vi "Facade.vi"(0 "Data In":T6, 2 "Display State In":T2={"Graph Visible Items"={"Plot Legend"=FALSE, "Scale Legend"=FALSE, "Graph Palette"=FALSE, "Cursor Legend"=FALSE, "X Scrollbar"=FALSE}, "View Table"=FALSE, "Table Visible Items"={"Vertical Scrollbar"=FALSE, "Horizontal Scrollbar"=FALSE, "Row Headers"=FALSE, "Column Headers"=FALSE, "Vertical Lines"=FALSE, "Horizontal Lines"=FALSE}, "Header Font"={"Font Name"="", "Size"=0, "Bold"=FALSE, "Italic"=FALSE, "Underline"=FALSE, "Strikeout"=FALSE, "Color"=0}, "Cell Font"={"Font Name"="", "Size"=0, "Bold"=FALSE, "Italic"=FALSE, "Underline"=FALSE, "Strikeout"=FALSE, "Color"=0}, "Description and Tip..."={"Description"="", "Tip"=""}, "Moveable Splitter Position"=0, "Measurement Cursor Configuration"={"relative to t0"={"enable relative time"=FALSE, "Relative times (DT)"=[], "color"=0}, "range"={"enable range"=FALSE, "T1"=0.0, "T2"=0.0, "Fixed interval (T2-T1)"=0.0, "T1 color"=0, "T2 color"=0, "enable shading"=FALSE}, "periodic"={"enable periodic"=FALSE, "First event (E1)"=0.0, "Number events (Ei)"=0, "Event spacing (s)"=0.0, "First color"=0, "Events color"=0}, "absolute timestamp"={"enable absolute"=FALSE, "Timestamps (TS)"=[], "color"=0}}, "X Increment"=0.0, "X Scale"={"Label Visible"=FALSE, "Label Text"="", "Time Mode"=enum."Relative", "Format String"=""}, "Y Scale"={"Label Visible"=FALSE, "Label Text"="", "Scaling"=enum."Engineering Units", "Format String"=""}, "Colors"={"background"=16777215, "major grid"=8355711, "minor grid"=12632256, "font"=0}, "Cursors"={"List"=[], "Tags"=[]}, "Plots"=[], "Plot Color Wheel"=[3381759, 32768, 982784, 4375295, 13827953, 13457919, 16757522, 4343295, 16728758, 12095254], "registered user events"=variant}, 3 "Container State":T5) -> (6 "Data Out":T6, 7 "Display State Out":T2={"Graph Visible Items"={"Plot Legend"=FALSE, "Scale Legend"=FALSE, "Graph Palette"=FALSE, "Cursor Legend"=FALSE, "X Scrollbar"=FALSE}, "View Table"=FALSE, "Table Visible Items"={"Vertical Scrollbar"=FALSE, "Horizontal Scrollbar"=FALSE, "Row Headers"=FALSE, "Column Headers"=FALSE, "Vertical Lines"=FALSE, "Horizontal Lines"=FALSE}, "Header Font"={"Font Name"="", "Size"=0, "Bold"=FALSE, "Italic"=FALSE, "Underline"=FALSE, "Strikeout"=FALSE, "Color"=0}, "Cell Font"={"Font Name"="", "Size"=0, "Bold"=FALSE, "Italic"=FALSE, "Underline"=FALSE, "Strikeout"=FALSE, "Color"=0}, "Description and Tip..."={"Description"="", "Tip"=""}, "Moveable Splitter Position"=0, "Measurement Cursor Configuration"={"relative to t0"={"enable relative time"=FALSE, "Relative times (DT)"=[], "color"=0}, "range"={"enable range"=FALSE, "T1"=0.0, "T2"=0.0, "Fixed interval (T2-T1)"=0.0, "T1 color"=0, "T2 color"=0, "enable shading"=FALSE}, "periodic"={"enable periodic"=FALSE, "First event (E1)"=0.0, "Number events (Ei)"=0, "Event spacing (s)"=0.0, "First color"=0, "Events color"=0}, "absolute timestamp"={"enable absolute"=FALSE, "Timestamps (TS)"=[], "color"=0}}, "X Increment"=0.0, "X Scale"={"Label Visible"=FALSE, "Label Text"="", "Time Mode"=enum."Relative", "Format String"=""}, "Y Scale"={"Label Visible"=FALSE, "Label Text"="", "Scaling"=enum."Engineering Units", "Format String"=""}, "Colors"={"background"=16777215, "major grid"=8355711, "minor grid"=12632256, "font"=0}, "Cursors"={"List"=[], "Tags"=[]}, "Plots"=[], "Plot Color Wheel"=[3381759, 32768, 982784, 4375295, 13827953, 13457919, 16757522, 4343295, 16728758, 12095254], "registered user events"=variant}, 8 "Action":T1)   [LabVIEW 2017, in "Waveforms with Cursors.xctl"]
doc: "This is the facade VI for the Spectral Graph with Measurement Cursors XControl.\nThe facade VI is only used within the context of the XControl."
uses:
  <vilib>/addons/_XControls/Waveforms with Cursors/Waveforms with Cursors.xctl
  <vilib>/addons/_XControls/Waveforms with Cursors/Controls/Data.ctl
  <vilib>/_xctls/Container State.ctl
  <vilib>/addons/_XControls/Waveforms with Cursors/Controls/State.ctl
  <vilib>/Utility/miscctls.llb/LVFontTypeDef.ctl
  <vilib>/addons/_XControls/Waveforms with Cursors/Controls/Waveform Cursor Configuration.ctl
  <vilib>/_xctls/Action.ctl
  <vilib>/addons/_XControls/Waveforms with Cursors/Controls/Refnums Typedef.ctl
  <vilib>/addons/_XControls/Waveforms with Cursors/Controls/Waveform XControl Events.ctl
  <vilib>/Utility/miscctls.llb/LVForegroundBackgroundColorsTypeDef.ctl
  <vilib>/measure/mamon.llb/Trigger Detection for 1 Channel.vi
  <vilib>/addons/_NISVFA/_Shared subVIs/Groups/SV Get By Measurement Type (sw trigger) (1 Ch).vi
  <vilib>/_xctls/XControlSupport.lvlib
  <vilib>/measure/NI_MAPro.lvlib
panel:
  out "plot names":string[](array[string])
  in  "Focus Boolean":bool
  out "Waveform Graph":waveform(sgl)[](graph)
  in  "View Table":bool=TRUE
  in  "Cursor Table":string[][](table)
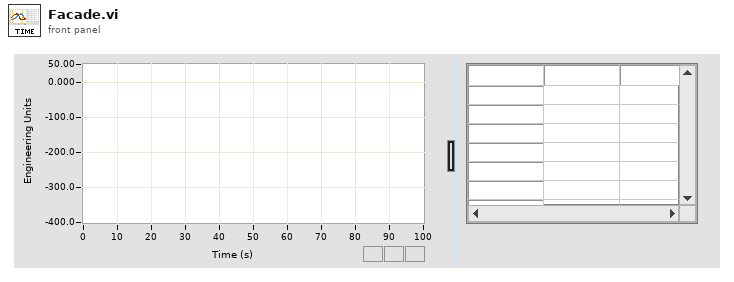
[diagram p1: front panel]
types:
  T1 = typedef "XControlSupport.lvlib/Action.ctl" = cluster{"Data Changed?":bool, "State Changed?":bool, "Action Name":string}
  T2 = typedef "Waveforms with Cursors.xctl/State.ctl" = cluster{"Graph Visible Items":cluster{"Plot Legend":bool, "Scale Legend":bool, "Graph Palette":bool, "Cursor Legend":bool, "X Scrollbar":bool}, "View Table":bool, "Table Visible Items":cluster{"Vertical Scrollbar":bool, "Horizontal Scrollbar":bool, "Row Headers":bool, "Column Headers":bool, "Vertical Lines":bool, "Horizontal Lines":bool}, "Header Font":T3, "Cell Font":T3, "Description and Tip...":cluster{"Description":string, "Tip":string}, "Moveable Splitter Position":i32, "Measurement Cursor Configuration":T4, "X Increment":dbl, "X Scale":cluster{"Label Visible":bool, "Label Text":string, "Time Mode":enum16{"Relative", "Absolute"}, "Format String":string}, "Y Scale":cluster{"Label Visible":bool, "Label Text":string, "Scaling":enum16{"Engineering Units", "Voltage"}, "Format String":string}, "Colors":cluster{"background":u32, "major grid":u32, "minor grid":u32, "font":u32}, "Cursors":cluster{"List":cluster{"Name":string, "Color":u32, "Style":i32, "Point Style":u8, "Name Visible":bool, "Allow Drag":bool, "Cursor Mode":u32, "Plot":i32, "Index":i32, "Position":cluster{"X":dbl, "Y":dbl}, "X Scale":u32, "Y Scale":u32, "Watch Plots":i32[], "Watch All Plots":bool, "Plot Area":i32, "Label Offset":cluster{"X":dbl, "Y":dbl}}[], "Tags":variant[]}, "Plots":cluster{"Name":string, "Line Color":u32, "Line Style":u8, "Line Width":u8, "Fill/Point Color":u32, "Point Style":u8, "Fill To":i16, "Interpolation":u8, "Anti-aliased":bool}[], "Plot Color Wheel":u32[], "registered user events":variant}
  T3 = typedef "LVFontTypeDef.ctl" = cluster{"Font Name":string, "Size":u16, "Bold":bool, "Italic":bool, "Underline":bool, "Strikeout":bool, "Color":u32}
  T4 = typedef "Waveforms with Cursors.xctl/Waveform Cursor Configuration.ctl" = cluster{"relative to t0":cluster{"enable relative time":bool, "Relative times (DT)":dbl[], "color":u32}, "range":cluster{"enable range":bool, "T1":dbl, "T2":dbl, "Fixed interval (T2-T1)":dbl, "T1 color":u32, "T2 color":u32, "enable shading":bool}, "periodic":cluster{"enable periodic":bool, "First event (E1)":dbl, "Number events (Ei)":i32, "Event spacing (s)":dbl, "First color":u32, "Events color":u32}, "absolute timestamp":cluster{"enable absolute":bool, "Timestamps (TS)":timestamp[], "color":u32}}
  T5 = typedef "XControlSupport.lvlib/Container State.ctl" = cluster{"Indicator?":bool, "Run Mode?":bool, " Refnum":refnum<vi>}
  T6 = typedef "Waveforms with Cursors.xctl/Data.ctl" = waveform(dbl)[]
  T7 = typedef "Waveforms with Cursors.xctl/Refnums Typedef.ctl" = cluster{"Splitters":cluster{"Moveable":refnum<vi>, "Locked":refnum<vi>}, "Panes":cluster{"Container":refnum<vi>, "Graph":refnum<vi>, "Table":refnum<vi>, "Fixed-Width":refnum<vi>}, "Controls":cluster{"WFGraph Refnum":refnum<vi>, "Table":refnum<vi>, "View Table":refnum<vi>, "Focus Boolean":refnum<vi>, "Plot Names":refnum<vi>}}
  T8 = typedef "Waveforms with Cursors.xctl/Waveform XControl Events.ctl" = string
  T9 = typedef "LVForegroundBackgroundColorsTypeDef.ctl" = cluster{"Foreground Color":u32, "Background Color":u32}
  T10 = cluster{"level":dbl, "slope":u16, "hysteresis":dbl}
  T11 = typedef "eventvkey.ctl" = enum16{"ASCII", "Enter", "Return", "Shift", "Ctrl", "Alt", "Cmd", "Opt", "Caps", "NumLock", "Clear", "Break", "Up", "Down", "Left", "Right", "Insert", "Delete", "Home", "End", "PageUp", "PageDown", "Escape", "Help", "Pause", "ScrollLock", "F1", "F2", "F3", "F4", "F5", "F6", "F7", "F8", "F9", "F10", "F11", "F12", "F13", "F14", "F15", "F16", "F17", "F18", "F19", "F20", "F21", "F22", "F23", "F24", "Play", "VolumeUp", "VolumeDown", "Mute", "Two Byte Char"}
  T12 = cluster{"Shift":bool, "Ctrl":bool, "Alt":bool, "Cmd":bool, "Opt":bool}
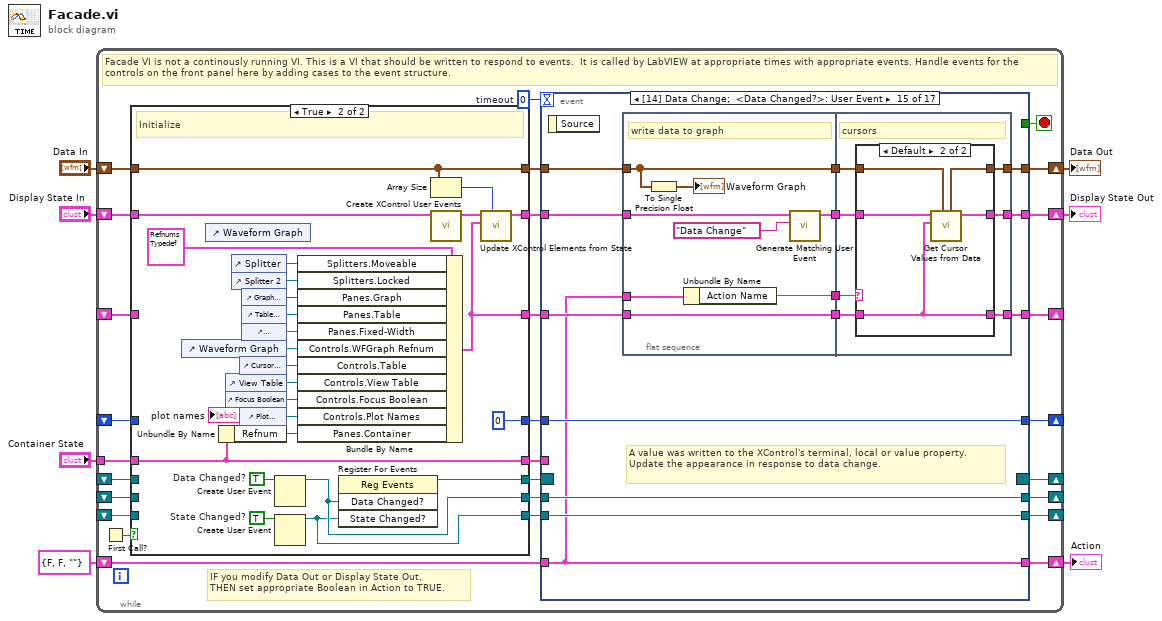
[diagram p0: block diagram]
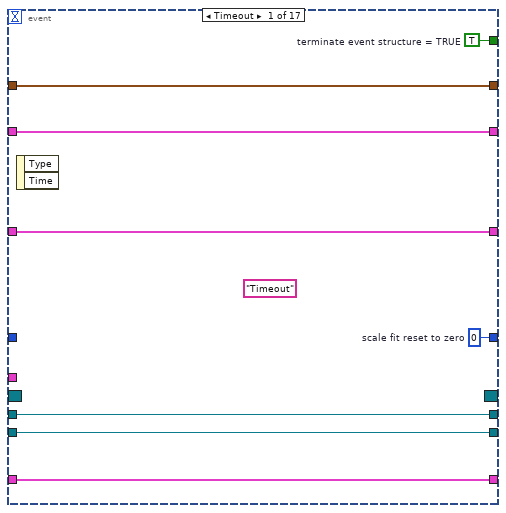
[diagram p3: hidden frame]
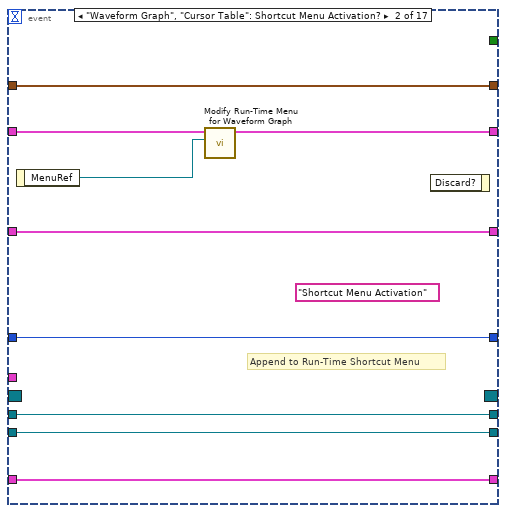
[diagram p4: hidden frame]
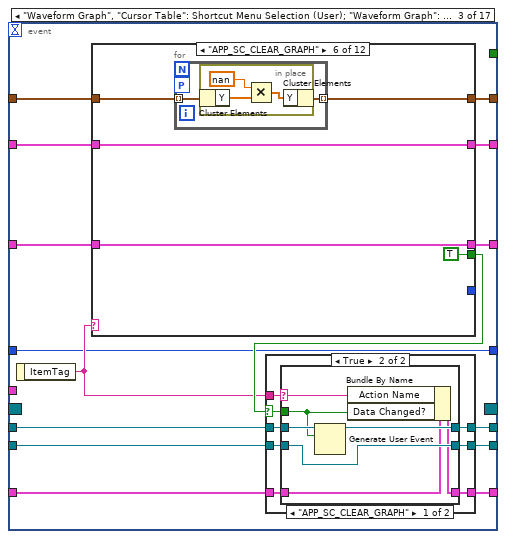
[diagram p5: hidden frame]
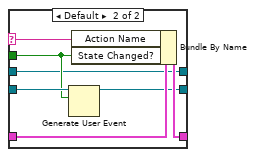
[diagram p7: hidden frame]
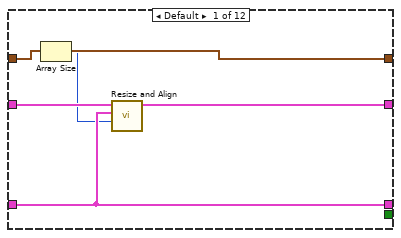
[diagram p8: hidden frame]
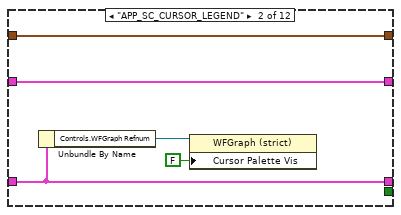
[diagram p9: hidden frame]
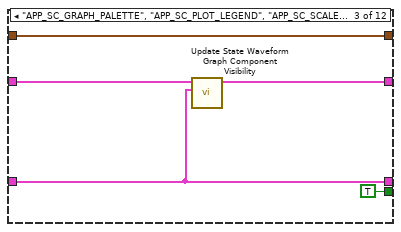
[diagram p10: hidden frame]
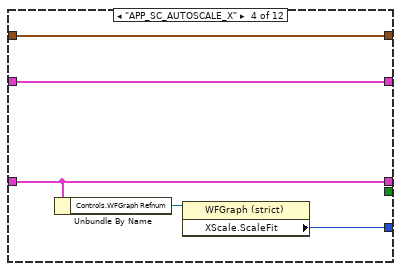
[diagram p11: hidden frame]
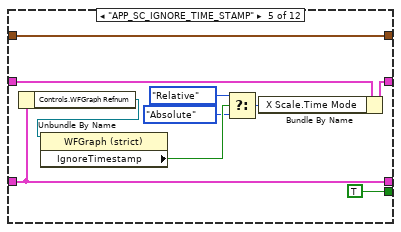
[diagram p12: hidden frame]
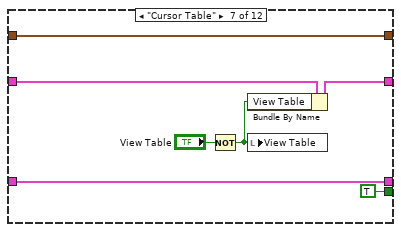
[diagram p13: hidden frame]
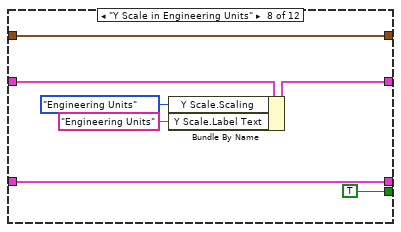
[diagram p14: hidden frame]
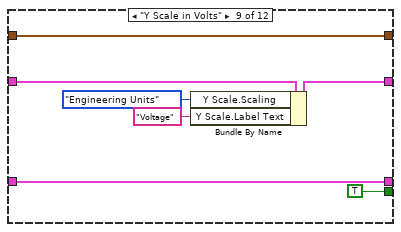
[diagram p15: hidden frame]
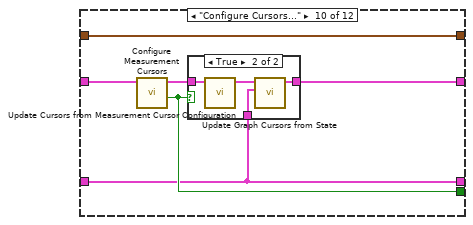
[diagram p16: hidden frame]
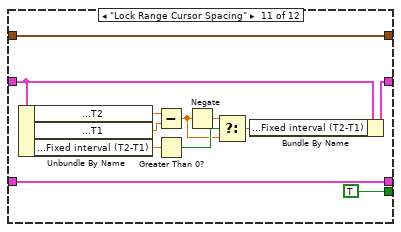
[diagram p18: hidden frame]
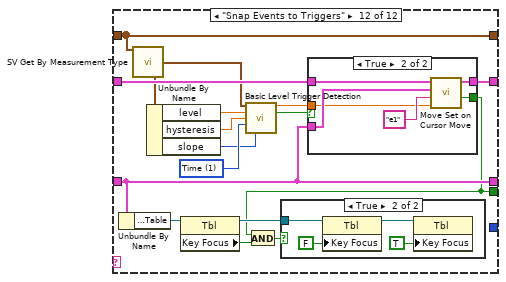
[diagram p19: hidden frame]
diagram:
  n1 = while {
    shift-right: [w15] -> w5
    shift-left: "Display State In" -> [w13]
    tunnel: "Container State" -> [w21]
    shift-right: [w33] -> w7
    shift-left: "Data In" -> [w8]
    shift-right: [w31] -> w2
    shift-left: T1 {"Data Changed?"=FALSE, "State Changed?"=FALSE, "Action Name"=""} ("Action") -> [w32]
    shift-right: [w28] -> _
    shift-left: _ -> [w26]
    shift-right: [w23] -> _
    shift-left: _ -> [w22]
    shift-right: [w27] -> _
    shift-left: _ -> [w24]
    shift-right: [w16] -> _
    shift-left: _ -> [w18]
    shift-right: [w11] -> _
    shift-left: _ -> [w12]
    stop <- w35 stop-if-true
    w34 = 0  # timeout
    # "IF you modify Data Out or Display State Out, \nTHEN set appropriate Boolean in Action to TRUE."
    # "Facade VI is not a continously running VI. This is a VI that should be written to respond to events.  It is called by LabVIEW at appropriate times with appropriate events. Handle events for the controls on the front panel here by adding cases to the event structure."
    n2 = First Call?() -> (First Call?: T/F=w25:bool)
    n3 = case shown="True" w25 {
      tunnel: [w43 w55] -> w17
      tunnel: [w42 w56] -> w30
      tunnel: [w41 w57] -> w29
      tunnel: w26 -> [w43 _]
      tunnel: w24 -> [w42 _]
      tunnel: w22 -> [w41 _]
      tunnel: w21 -> [w39 w51]
      tunnel: [w39 w51] -> w20
      tunnel: [w40 w49] -> w19
      tunnel: w18 -> [w40 _]
      tunnel: [w38 w50] -> w14
      tunnel: w13 -> [w38 w48]
      tunnel: [w37 u8 0 ("Scale Fit")] -> w10
      tunnel: w12 -> [w37 _]
      tunnel: [w36 w45] -> w9
      tunnel: w8 -> [w36 w45]
      frame False {
        # "Continue"
      }
      frame True {
        w68 = TRUE  # State Changed?
        w67 = TRUE  # Data Changed?
        # "Initialize"
        n4 = control-ref of="Waveform Graph"() -> (w63:refnum<vi>)
        n5 = control-ref of="Waveform Graph"() -> ()  [unwired: 1 out]
        n6 = Unbundle By Name(w51) -> ("Refnum"=w53:refnum<vi>)
        n7 = control-ref of="View Table"() -> (w61:refnum<vi>)
        n8 = control-ref of="Focus Boolean"() -> (w54:refnum<vi>)
        n9 = control-ref of="Splitter"() -> (w60:refnum<vi>)
        n10 = control-ref of="Splitter 2"() -> (w59:refnum<vi>)
        n11 = control-ref of="Cursor Table"() -> (w62:refnum<vi>)
        n12 = control-ref of="Plot Names"() -> (w52:refnum<vi>)
        n13 = control-ref of="Graph Pane"() -> (w58:refnum<vi>)
        n14 = control-ref of="Table Pane"() -> (w65:refnum<vi>)
        n15 = control-ref of="Fixed-Width Pane"() -> (w64:refnum<vi>)
        n16 = Create User Event(user event datatype=w67) -> (user event=w57:refnum<user-event>)  [unwired: 1 in, 1 out]
        n17 = Create User Event(user event datatype=w68) -> (user event=w56:refnum<user-event>)  [unwired: 1 in, 1 out]
        n18 = Bundle By Name(cluster=T7 {"Splitters"={"Moveable"=refnum, "Locked"=refnum}, "Panes"={"Container"=refnum, "Graph"=refnum, "Table"=refnum, "Fixed-Width"=refnum}, "Controls"={"WFGraph Refnum"=refnum, "Table"=refnum, "View Table"=refnum, "Focus Boolean"=refnum, "Plot Names"=refnum}} ("Refnums for Resizing and Alignment"), "Splitters.Moveable"=w60, "Splitters.Locked"=w59, "Panes.Graph"=w58, "Panes.Table"=w65, "Panes.Fixed-Width"=w64, "Controls.WFGraph Refnum"=w63, "Controls.Table"=w62, "Controls.View Table"=w61, "Controls.Focus Boolean"=w54, "Controls.Plot Names"=w52, "Panes.Container"=w53) -> (w49:T7)
        n19 = register-events(w57, w56) -> (reference out=w55:refnum<event-registration>)  [unwired: 2 in, 1 out]
        n20 = Array Size(array=w45) -> (size(s)=w44:i32)
        n21 = call <vilib>:"Create XControl User Events.vi"("Display State In in"=w48) -> ("Display State In out"=w47:T2)  [unwired: 9 in, 1 out]
        n22 = call <vilib>:"Update XControl Elements from State.vi"("number of channels"=w44, "Refnums for FP Objects"=w49, "State in"=w47) -> ("State out"=w50:T2)  [unwired: 8 in]
      }
    }
    n23 = event shown="[14] Data Change;  <Data Changed?>: User Event" {
      selector: w17 -> [_ _ _ _ _ _ _ _ _ _ _ _ _ _ _ _ _]
      dyn-events: [_ _ _ _ _ _ _ _ _ _ _ _ _ _ _ _ _] -> w28
      timeout: w34 -> [_ _ _ _ _ _ _ _ _ _ _ _ _ _ _ _ _]
      tunnel: w14 -> [w70 w78 w100 w245 w268 w285 w310 w337 w352 w367 w408 w446 w480 w498 w537 w566 w578]
      tunnel: [w70 w79 w88 w244 w263 w284 w309 w321 w351 w359 w399 w437 w475 w497 w531 w566 w578] -> w15
      tunnel: [w76 _ _ _ _ _ _ _ _ _ _ _ _ _ _ _ _] -> w35
      tunnel: w20 -> [_ _ _ _ _ _ _ _ _ _ _ _ _ _ _ w576 w584]
      tunnel: w9 -> [w74 w85 w90 w238 w272 w302 w319 w338 w356 w377 w417 w455 w485 w487 w535 w575 w583]
      tunnel: [w74 w85 w86 w238 w272 w302 w319 w338 w356 w377 w417 w455 w485 w487 w538 w575 w583] -> w33
      tunnel: [w75 w84 w98 w248 w271 w298 w315 w335 w355 w375 w415 w453 w484 w502 w528 w574 w582] -> w31
      tunnel: w32 -> [w75 w84 w99 w248 w271 w299 w316 w336 w355 w376 w416 w454 w484 w494 w528 w574 w582]
      tunnel: w19 -> [w71 w81 w93 w242 w269 w291 w311 w324 w350 w365 w406 w445 w481 w499 w536 w567 w579]
      tunnel: w29 -> [w73 w83 w94 w246 w265 w297 w314 w330 w353 w371 w411 w449 w482 w501 w540 w571 w581]
      tunnel: w30 -> [w72 w82 w97 w247 w264 w296 w313 w333 w354 w374 w414 w452 w483 w488 w539 w570 w580]
      tunnel: [w72 w82 w96 w247 w264 w295 w312 w332 w354 w373 w413 w451 w483 w489 w539 w570 w580] -> w27
      tunnel: [w73 w83 w95 w246 w265 w297 w314 w331 w353 w372 w412 w450 w482 w500 w540 w571 w581] -> w23
      tunnel: [w71 w81 w92 w243 w269 w291 w311 w324 w350 w365 w406 w445 w481 w495 w530 w567 w579] -> w16
      tunnel: [w69 w77 w87 w239 w261 w281 w307 w320 w349 w357 w398 w436 w474 w491 w529 w565 w577] -> w11
      tunnel: w10 -> [_ w77 w87 _ w262 w281 w307 w320 w349 w357 w398 w436 w474 w491 w529 w565 w577]
      event Timeout {
        w69 = u8 0  # scale fit reset to zero
        (unwired) "Timeout"
        w76 = TRUE  # terminate event structure = TRUE
        n24 = event-data() -> ()  [unwired: 1 in, 2 out]
      }
      event "Waveform Graph", "Cursor Table": Shortcut Menu Activation? {
        (unwired) "Shortcut Menu Activation"
        # "Append to Run-Time Shortcut Menu"
        n25 = event-data() -> ("MenuRef"=w80:refnum<k9>)  [unwired: 1 in]
        n26 = call <vilib>:"Modify Run-Time Menu for Waveform Graph.vi"("Menu in"=w80, "Display State In"=w78) -> ("Display State out"=w79:T2)  [unwired: 9 in]
        n27 = event-data() -> ()  [unwired: 2 in, 1 out]
      }
      event "Waveform Graph", "Cursor Table": Shortcut Menu Selection (User); "Waveform Graph": Shortcut Menu Selection (App) {
        n28 = event-data() -> ("ItemTag"=w89:string)  [unwired: 1 in]
        n29 = case shown="\"APP_SC_CLEAR_GRAPH\"" w89 {
          tunnel: w100 -> [w130 w135 w139 w145 w154 w160 w170 w176 w183 w192 w208 w225]
          tunnel: [w129 w135 w138 w145 w153 w160 w169 w175 w182 w190 w207 w226] -> w88
          tunnel: [_ _ TRUE ("state changed") _ TRUE ("state changed") TRUE ("state changed") TRUE ("state changed") TRUE ("state changed") TRUE ("state changed") w189 TRUE ("state changed") w219] -> w91
          tunnel: w93 -> [w128 w133 w137 w144 w152 w159 w172 w178 w185 w188 w209 w224]
          tunnel: [w128 w133 w137 w144 w152 w159 w172 w178 w185 w188 w209 w224] -> w92
          tunnel: w90 -> [w127 w134 w136 w141 w146 w158 w166 w173 w180 w187 w198 w218]
          tunnel: [_ _ _ w142 _ _ _ _ _ _ _ _] -> _
          tunnel: [w127 w134 w136 w141 w146 w157 w166 w173 w180 w187 w198 w218] -> w86
          frame Default {
            n30 = Array Size(array=w127) -> (size(s)=w126:i32)
            n31 = call <vilib>:"Resize and Align.vi"("number of channels"=w126, "Refnums for Resizing and Alignment"=w128, "State in"=w130) -> ("State out"=w129:T2)  [unwired: 7 in, 1 out]
          }
          frame "APP_SC_CURSOR_LEGEND" {
            n32 = Unbundle By Name(w133) -> ("Controls.WFGraph Refnum"=w132:refnum<vi>)
            n33 = property class="WFGraph (strict)"(reference=w132, "Cursor Palette Vis"=FALSE ("Cursor Legend Visible")) -> ()  [unwired: 1 in, 2 out]
          }
          frame "APP_SC_GRAPH_PALETTE", "APP_SC_PLOT_LEGEND", "APP_SC_SCALE_LEGEND", "APP_SC_X_SCALE", "APP_SC_X_SCROLLBAR", "APP_SC_Y_SCALE" {
            n34 = call <vilib>:"Update State Waveform Graph Component Visibility.vi"("Refnums for FP Objects"=w137, "State in"=w139) -> ("State out"=w138:T2)  [unwired: 9 in]
          }
          frame "APP_SC_AUTOSCALE_X" {
            n35 = Unbundle By Name(w144) -> ("Controls.WFGraph Refnum"=w143:refnum<vi>)
            n36 = property class="WFGraph (strict)"(reference=w143) -> ("XScale.ScaleFit"=w142:u8)  [unwired: 1 in, 2 out]
          }
          frame "APP_SC_IGNORE_TIME_STAMP" {
            n37 = Unbundle By Name(w152) -> ("Controls.WFGraph Refnum"=w151:refnum<vi>)
            n38 = property class="WFGraph (strict)"(reference=w151) -> ("IgnoreTimestamp"=w150:bool)  [unwired: 1 in, 2 out]
            n39 = Select(t=enum16{"Relative", "Absolute"}."Relative" ("X Scale.Time Mode"), s=w150, f=enum16{"Relative", "Absolute"}."Absolute") -> (s? t:f=w147:enum16{"Relative", "Absolute"})
            n40 = Bundle By Name(cluster=w154, "X Scale.Time Mode"=w147) -> (w153:T2)
          }
          frame "APP_SC_CLEAR_GRAPH" {
            n41 = for {
              tunnel: w158 -> [w162] mode=indexing
              tunnel: [w161] -> w157 mode=indexing
              workers-P: _ -> [_]
              n42 = in-place {
                n43 = in-place-cluster #1(w162) -> ("Y"=w164:dbl[])
                n44 = Multiply(x=nan, y=w164) -> (x*y=w163:dbl[])
                n45 = in-place-cluster #1("Y"=w163) -> (w161:waveform(dbl))
              }
            }
          }
          frame "Cursor Table" {
            n46 = Not(x="View Table") -> (.not. x?=w168:bool)
            n47 = Bundle By Name(cluster=w170, "View Table"=w168) -> (w169:T2)
            n48 = local write "View Table"(w168) -> ()
          }
          frame "Y Scale in Engineering Units" {
            n49 = Bundle By Name(cluster=w176, "Y Scale.Scaling"=enum16{"Engineering Units", "Voltage"}."Engineering Units", "Y Scale.Label Text"="Engineering Units") -> (w175:T2)
          }
          frame "Y Scale in Volts" {
            n50 = Bundle By Name(cluster=w183, "Y Scale.Scaling"=enum16{"Engineering Units", "Voltage"}."Engineering Units", "Y Scale.Label Text"="Voltage") -> (w182:T2)
          }
          frame "Configure Cursors..." {
            n51 = call <vilib>:"Configure Measurement Cursors.vi"("State in"=w192) -> ("OK"=w189:bool, "State out"=w191:T2)  [unwired: 9 in]
            n52 = case shown="True" w189 {
              tunnel: w191 -> [w193 w197]
              tunnel: [w193 w195] -> w190
              tunnel: w188 -> [_ w194]
              frame False {
              }
              frame True {
                n53 = call <vilib>:"Update Cursors from Measurement Cursor Configuration.vi"("State in"=w197) -> ("State out"=w196:T2)  [unwired: 10 in]
                n54 = call <vilib>:"Update Graph Cursors from State.vi"("Refnums for FP Objects"=w194, "State in"=w196) -> ("State out"=w195:T2)  [unwired: 9 in]
              }
            }
          }
          frame "Lock Range Cursor Spacing" {
            n55 = Unbundle By Name(w208) -> ("Measurement Cursor Configuration.range.T2"=w206:dbl, "Measurement Cursor Configuration.range.T1"=w205:dbl, "Measurement Cursor Configuration.range.Fixed interval (T2-T1)"=w204:dbl)
            n56 = Subtract(x=w206, y=w205) -> (x-y=w200:dbl)
            n57 = Greater Than 0?(x=w204) -> (x > 0?=w203:bool)
            n58 = Negate(x=w200) -> (-x=w202:dbl)
            n59 = Select(t=w202, s=w203, f=w200) -> (s? t:f=w201:dbl)
            n60 = Bundle By Name(cluster=w208, "Measurement Cursor Configuration.range.Fixed interval (T2-T1)"=w201) -> (w207:T2)
          }
          frame "Snap Events to Triggers" {
            w215 = u16 1 items=["Index", "Time"] ("location mode")
            n61 = Unbundle By Name(w224) -> ("Controls.Table"=w223:refnum<vi>)
            n62 = call-poly <vilib>:"SV Get By Measurement Type.vi"("scaled signals [EU]"=w218) -> ("trigger channel"=w217:waveform(dbl), "level trigger configuration"=w213:T10)  [unwired: 8 in, 5 out]
            n63 = Unbundle By Name(w213) -> ("level"=w212:dbl, "hysteresis"=w211:dbl, "slope"=w210:u16)
            n64 = property class="Tbl"(reference=w223) -> (reference out=w222:refnum<vi>, "Key Focus"=w221:bool)  [unwired: 1 in, 1 out]
            n65 = call-poly <vilib>:"Basic Level Trigger Detection.vi"("signal in"=w217, "level"=w212, "hysteresis"=w211, "location mode"=w215, "trigger slope"=w210) -> ("trigger location"=w214:dbl, "trigger detected?"=w216:bool)  [unwired: 8 in, 1 out]
            n66 = case shown="True" w216 {
              tunnel: [w231 w237] -> w226
              tunnel: w225 -> [w231 w236]
              tunnel: w224 -> [_ w235]
              tunnel: [_ w233] -> w219
              tunnel: w214 -> [_ w232]
              frame False {
              }
              frame True {
                n67 = call <vilib>:"Move Set on Cursor Move.vi"("Cursor.Position.X"=w232, "Cursor Name"="e1", "Refnums for Resizing and Alignment"=w235, "Display State In"=w236) -> ("state changed"=w233:bool, "Display State Out"=w237:T2)  [unwired: 6 in]
              }
            }
            n68 = And(x=w219, y=w221) -> (x .and. y?=w220:bool)
            n69 = case shown="True" w220 {
              tunnel: w222 -> [_ w229]
              frame False {
              }
              frame True {
                n70 = property class="Tbl"(reference=w229, "Key Focus"=FALSE) -> (reference out=w228:refnum<vi>)  [unwired: 1 in, 1 out]
                n71 = property class="Tbl"(reference=w228, "Key Focus"=TRUE) -> ()  [unwired: 1 in, 2 out]
              }
            }
          }
        }
        n72 = case shown="True" w91 {
          selector: w91 -> [_ w107]
          tunnel: w99 -> [w103 w111]
          tunnel: [w103 w110] -> w98
          tunnel: w89 -> [_ w106]
          tunnel: w97 -> [w102 w109]
          tunnel: [w102 w108] -> w96
          tunnel: [w101 w105] -> w95
          tunnel: w94 -> [w101 w104]
          frame False {
          }
          frame True {
            n73 = case shown="\"APP_SC_CLEAR_GRAPH\"" w106 {
              selector: w106 -> [w112 w120]
              tunnel: w111 -> [w114 w125]
              tunnel: [w113 w124] -> w110
              tunnel: w109 -> [w118 w123]
              tunnel: [w118 w122] -> w108
              tunnel: w107 -> [w115 w121]
              tunnel: [w116 w119] -> w105
              tunnel: w104 -> [w117 w119]
              frame "APP_SC_CLEAR_GRAPH" {
                n74 = Generate User Event(user event=w117, event data cluster=w115) -> (user event out=w116:refnum<user-event>)  [unwired: 2 in, 1 out]
                n75 = Bundle By Name(cluster=w114, "Action Name"=w112, "Data Changed?"=w115) -> (w113:T1)
              }
              frame Default {
                n76 = Generate User Event(user event=w123, event data cluster=w121) -> (user event out=w122:refnum<user-event>)  [unwired: 2 in, 1 out]
                n77 = Bundle By Name(cluster=w125, "Action Name"=w120, "State Changed?"=w121) -> (w124:T1)
              }
            }
          }
        }
      }
      event "Waveform Graph": Autoscale Range Change {
        n78 = event-data() -> ("Kind"=w240:enum16{"X-Scale", "Y-Scale", "Z-Scale"}, "ScaleRef"=w241:refnum<vi>)  [unwired: 1 in]
        n79 = property class="GrphScl"(reference=w241) -> ("ScaleFit"=w239:u8)  [unwired: 1 in, 2 out]
        n80 = case shown="\"Y-Scale\"" w240 {
          tunnel: w245 -> [w250 w255]
          tunnel: [w250 w254] -> w244
          tunnel: [w249 w253] -> w243
          tunnel: w242 -> [w249 w252]
          tunnel: w239 -> [_ w251]
          frame "X-Scale", Default {
          }
          frame "Y-Scale" {
            n81 = case shown="1, 2" w251 {
              tunnel: w255 -> [w257 w260]
              tunnel: w252 -> [w256 w258]
              tunnel: [w257 w259] -> w254
              tunnel: [w256 w258] -> w253
              frame 0, Default {
                # "YScaleFit\nManual"
              }
              frame 1, 2 {
                # "YScaleFit\nAuto"
                n82 = call <vilib>:"Adjust Cursor Y Position to Maintain Label Placement.vi"("Refnums for Resizing and Alignment"=w258, "Display State In"=w260) -> ("Display State Out"=w259:T2)  [unwired: 9 in]
              }
            }
          }
        }
      }
      event "Waveform Graph": Scale Range Change {
        (unwired) "Scale Range Change"
        # "this tells us if the scale range changed due to autoscale being set"
        n83 = event-data() -> ("Kind"=w267:enum16{"X-Scale", "Y-Scale", "Z-Scale"}, "ScaleRef"=w270:refnum<vi>)  [unwired: 1 in]
        n84 = case shown="0" w262 {
          selector: w262 -> [_ w274]
          tunnel: w270 -> [_ w276]
          tunnel: [_ w275] -> w266
          tunnel: [u8 0 ("Scale Fit") w274] -> w261
          frame Default {
          }
          frame 0 {
            n85 = property class="GrphScl"(reference=w276, "ScaleFit"=w274) -> (error out=w275:errorcluster)  [unwired: 1 in, 1 out]
          }
        }
        n86 = case shown="\"Y-Scale\"" w267 {
          tunnel: w269 -> [_ w280]
          tunnel: w268 -> [w277 w279]
          tunnel: [w277 w278] -> w263
          tunnel: w266 -> [_ _]
          frame Default {
          }
          frame "Y-Scale" {
            n87 = call <vilib>:"Adjust Cursor Y Position to Maintain Label Placement.vi"("Refnums for Resizing and Alignment"=w280, "Display State In"=w279) -> ("Display State Out"=w278:T2)  [unwired: 9 in]
          }
        }
      }
      event Pane Size {
        w293 = 10  # width - hidden splitter position
        w300 = TRUE
        n88 = event-data() -> ()  [unwired: 1 in, 6 out]
        n89 = Unbundle By Name(w291) -> ("Panes.Container"=w289:refnum<vi>, "Splitters.Moveable"=w290:refnum<vi>)
        n90 = property class="Ctl"(reference=w289) -> ("Width"=w294:u32)  [unwired: 1 in, 2 out]
        n91 = property class="Splitter"(reference=w290) -> ("Position"=w282:i32)  [unwired: 1 in, 2 out]
        n92 = Generate User Event(user event=w296, event data cluster=w300) -> (user event out=w295:refnum<user-event>)  [unwired: 2 in, 1 out]
        n93 = To Long Integer(number=w294) -> (32bit integer=w292:i32)
        n94 = Bundle By Name(cluster=w299, "Action Name"="Resize", "State Changed?"=w300) -> (w298:T1)
        n95 = Unbundle By Name(w285) -> ("View Table"=w286:bool)
        n96 = Subtract(x=w292, y=w293) -> (x-y=w288:i32)
        n97 = Not Equal?(x=w288, y=w282) -> (x != y?=w287:bool)
        n98 = And(x=w286, y=w287) -> (x .and. y?=w283:bool)
        n99 = case shown="True" w283 {
          tunnel: w285 -> [w303 w306]
          tunnel: [w303 w305] -> w284
          tunnel: w282 -> [_ w304]
          frame False {
          }
          frame True {
            n100 = Bundle By Name(cluster=w306, "Moveable Splitter Position"=w304) -> (w305:T2)
          }
        }
      }
      event "View Table": Value Change {
        w317 = TRUE
        n101 = event-data() -> ("NewVal"=w308:bool)  [unwired: 1 in]
        n102 = Bundle By Name(cluster=w310, "View Table"=w308) -> (w309:T2)
        n103 = Generate User Event(user event=w313, event data cluster=w317) -> (user event out=w312:refnum<user-event>)  [unwired: 2 in, 1 out]
        n104 = Bundle By Name(cluster=w316, "Action Name"="View Table Value Change", "State Changed?"=w317) -> (w315:T1)
      }
      event "Waveform Graph": Cursor Move; "Waveform Graph": Cursor Grab {
        n105 = event-data() -> ("CursRef"=w328:refnum<vi>, "CursLoc"=w329:cluster{"X":dbl, "Y":dbl})  [unwired: 1 in]
        n106 = property class="Curs"(reference=w328) -> ("Cursor Name"=w327:string)  [unwired: 1 in, 2 out]
        n107 = Unbundle By Name(w329) -> ("X"=w326:dbl)
        n108 = call <vilib>:"Move Set on Cursor Move.vi"("Cursor.Position.X"=w326, "Cursor Name"=w327, "Refnums for Resizing and Alignment"=w324, "Display State In"=w337) -> ("state changed"=w325:bool, "Display State Out"=w321:T2)  [unwired: 6 in]
        n109 = Unbundle By Name(w324) -> ("Controls.Focus Boolean"=w323:refnum<vi>)
        n110 = case shown="True" w325 {
          selector: w325 -> [_ w344]
          tunnel: w336 -> [w341 w348]
          tunnel: [w341 w347] -> w335
          tunnel: "Cursor Move" -> [_ w346]
          tunnel: w333 -> [w340 w345]
          tunnel: [w340 w343] -> w332
          tunnel: [w339 w342] -> w331
          tunnel: w330 -> [w339 w342]
          frame False {
          }
          frame True {
            n111 = Generate User Event(user event=w345, event data cluster=w344) -> (user event out=w343:refnum<user-event>)  [unwired: 2 in, 1 out]
            n112 = Bundle By Name(cluster=w348, "Action Name"=w346, "State Changed?"=w344) -> (w347:T1)
          }
        }
        n113 = property class="Bool (strict)"(reference=w323, "Key Focus"=TRUE) -> ()  [unwired: 1 in, 2 out]
      }
      event "Waveform Graph": Plot Attribute Change {
        n114 = event-data() -> ()  [unwired: 1 in, 2 out]
        n115 = call <vilib>:"Update State Plot Properties.vi"("Refnums for FP Objects"=w350, "State in"=w352) -> ("State out"=w351:T2)  [unwired: 9 in]
      }
      event "Cursor Table": Value Change {
        n116 = event-data() -> ("OldVal"=w360:string[][], "CtlRef"=w361:refnum<vi>)  [unwired: 1 in]
        n117 = call <vilib>:"Verify New Value is Valid Numeric X Value.vi"("OldVal"=w360, "NewVal"="Cursor Table", "Refnums for Resizing and Alignment"=w365, "State in"=w367) -> ("X position"=w362:dbl, "cursor name"=w363:string, "Refnums for Resizing and Alignment out"=w364:T7, "State out"=w366:T2, "valid X change"=w369:bool)  [unwired: 3 in]
        n118 = case shown="True" w369 {
          selector: w369 -> [w378 _]
          tunnel: w364 -> [_ w385]
          tunnel: w366 -> [w379 w384]
          tunnel: [w379 w383] -> w359
          tunnel: [w378 w382] -> w368
          tunnel: w363 -> [_ w381]
          tunnel: w362 -> [_ w380]
          frame False {
          }
          frame True {
            n119 = call <vilib>:"Move Set on Cursor Move.vi"("Cursor.Position.X"=w380, "Cursor Name"=w381, "Refnums for Resizing and Alignment"=w385, "Display State In"=w384) -> ("state changed"=w382:bool, "Display State Out"=w383:T2)  [unwired: 6 in]
          }
        }
        n120 = case shown="True" w368 {
          selector: w368 -> [_ w391]
          tunnel: w376 -> [w390 w397]
          tunnel: [w390 w396] -> w375
          tunnel: "Cursor Move" -> [_ w395]
          tunnel: w374 -> [w389 w394]
          tunnel: [w389 w393] -> w373
          tunnel: [w388 w392] -> w372
          tunnel: w371 -> [w388 w392]
          tunnel: w361 -> [w387 _]
          tunnel: w360 -> [w386 _]
          frame False {
            n121 = property on="Property Node" class="Tbl (strict)"(reference=w387, "Value"=w386) -> ()  [unwired: 1 in, 2 out]
          }
          frame True {
            n122 = Bundle By Name(cluster=w397, "State Changed?"=w391, "Action Name"=w395) -> (w396:T1)
            n123 = Generate User Event(user event=w394, event data cluster=w391) -> (user event out=w393:refnum<user-event>)  [unwired: 2 in, 1 out]
          }
        }
      }
      event "Cursor Table", "Focus Boolean": Key Down? {
        n124 = event-data() -> ("VKey"=w409:T11, "PlatMods"=w402:T12)  [unwired: 1 in]
        n125 = call <vilib>:"Update XControl Based on Arrow Key Input.vi"("PlatMods"=w402, "VKey"=w409, "Refnums for Resizing and Alignment in"=w406, "display state in"=w408) -> ("Position.X"=w403:dbl, "selected cursor"=w404:string, "Refnums for Resizing and Alignment out"=w405:T7, "display state out"=w407:T2, "discard?"=w400:bool)  [unwired: 3 in]
        n126 = case shown="True" w400 {
          selector: w400 -> [w418 _]
          tunnel: w405 -> [_ w425]
          tunnel: w407 -> [w419 w424]
          tunnel: [w419 w423] -> w399
          tunnel: [w418 w422] -> w401
          tunnel: w404 -> [_ w421]
          tunnel: w403 -> [_ w420]
          frame False {
          }
          frame True {
            n127 = call <vilib>:"Move Set on Cursor Move.vi"("Cursor.Position.X"=w420, "Cursor Name"=w421, "Refnums for Resizing and Alignment"=w425, "Display State In"=w424) -> ("state changed"=w422:bool, "Display State Out"=w423:T2)  [unwired: 6 in]
          }
        }
        n128 = case shown="True" w401 {
          selector: w401 -> [_ w429]
          tunnel: w416 -> [w428 w435]
          tunnel: [w428 w434] -> w415
          tunnel: "Cursor Move" -> [_ w433]
          tunnel: w414 -> [w427 w432]
          tunnel: [w427 w431] -> w413
          tunnel: [w426 w430] -> w412
          tunnel: w411 -> [w426 w430]
          frame False {
          }
          frame True {
            n129 = Bundle By Name(cluster=w435, "State Changed?"=w429, "Action Name"=w433) -> (w434:T1)
            n130 = Generate User Event(user event=w432, event data cluster=w429) -> (user event out=w431:refnum<user-event>)  [unwired: 2 in, 1 out]
          }
        }
        n131 = event-data("Discard?"=w400) -> ()  [unwired: 1 in, 1 out]
      }
      event "Cursor Table", "Focus Boolean": event type 3.0.x8000000b {
        n132 = event-data() -> ("VKey"=w442:T11, "PlatMods"=w443:T12)  [unwired: 1 in]
        n133 = call <vilib>:"Update XControl Based on Arrow Key Input.vi"("PlatMods"=w443, "VKey"=w442, "Refnums for Resizing and Alignment in"=w445, "display state in"=w446) -> ("Position.X"=w438:dbl, "selected cursor"=w439:string, "Refnums for Resizing and Alignment out"=w440:T7, "display state out"=w441:T2, "discard?"=w444:bool)  [unwired: 3 in]
        n134 = case shown="True" w444 {
          selector: w444 -> [w456 _]
          tunnel: w440 -> [_ w463]
          tunnel: w441 -> [w457 w462]
          tunnel: [w457 w461] -> w437
          tunnel: [w456 w460] -> w447
          tunnel: w439 -> [_ w459]
          tunnel: w438 -> [_ w458]
          frame False {
          }
          frame True {
            n135 = call <vilib>:"Move Set on Cursor Move.vi"("Cursor.Position.X"=w458, "Cursor Name"=w459, "Refnums for Resizing and Alignment"=w463, "Display State In"=w462) -> ("state changed"=w460:bool, "Display State Out"=w461:T2)  [unwired: 6 in]
          }
        }
        n136 = case shown="True" w447 {
          selector: w447 -> [_ w467]
          tunnel: w454 -> [w466 w473]
          tunnel: [w466 w472] -> w453
          tunnel: "Cursor Move" -> [_ w471]
          tunnel: w452 -> [w465 w470]
          tunnel: [w465 w469] -> w451
          tunnel: [w464 w468] -> w450
          tunnel: w449 -> [w464 w468]
          frame False {
          }
          frame True {
            n137 = Bundle By Name(cluster=w473, "State Changed?"=w467, "Action Name"=w471) -> (w472:T1)
            n138 = Generate User Event(user event=w470, event data cluster=w467) -> (user event out=w469:refnum<user-event>)  [unwired: 2 in, 1 out]
          }
        }
        n139 = event-data("Discard?"=w444) -> ()  [unwired: 1 in, 1 out]
      }
      event "Cursor Table": Mouse Down {
        (unwired) "Cursor Table Mouse Down" ("ItemTag")
        n140 = event-data() -> ("Coords.Horizontal"=w479:i32, "Coords.Vertical"=w478:i32)  [unwired: 1 in]
        n141 = Bundle By Name(cluster=cluster{"horizontal":i32, "vertical":i32} {"horizontal"=0, "vertical"=0} ("Point"), "horizontal"=w479, "vertical"=w478) -> (w476:cluster{"horizontal":i32, "vertical":i32})
        n142 = call <vilib>:"Set Active Cursor from Table.vi"("Point"=w476, "Refnums for Resizing and Alignment"=w481, "Display State In"=w480) -> ("Display State Out"=w475:T2)  [unwired: 8 in]
      }
      event Display State Change; User Event {
        w492 = T8 "Display State Change"
        # "Display State Change is result of dropping a new instance of this XControl, copying, undoing an operation or executing a custom property or method on this XControl. Update the appearance accordingly."
        n143 = event-data() -> ()  [unwired: 1 in, 3 out]
        n144 = Unbundle By Name(w494) -> ("Action Name"=w493:string)
        n145 = Array Size(array=w487) -> (size(s)=w486:i32)
        n146 = case shown="Default" w493 {
          selector: w493 -> [_ w519]
          tunnel: w499 -> [w514 w520]
          tunnel: w498 -> [w515 w522]
          tunnel: [w515 w521] -> w496
          tunnel: [w514 w520] -> w495
          tunnel: [TRUE w517] -> w490
          tunnel: w486 -> [_ w516]
          frame "Cursor Move" {
          }
          frame Default {
            n147 = call <vilib>:"Update Graph Cursors from State.vi"("Refnums for FP Objects"=w520, "State in"=w522) -> ("State out"=w523:T2)  [unwired: 9 in]
            n148 = call <vilib>:"Set Graph Scale Properties.vi"("Refnums in"=w520, "Display State In"=w523) -> ("Display State out"=w525:T2)  [unwired: 9 in]
            n149 = call <vilib>:"Resize and Align.vi"("number of channels"=w516, "Refnums for Resizing and Alignment"=w520, "State in"=w525) -> ("State out"=w524:T2)  [unwired: 7 in, 1 out]
            n150 = Not Equal?(x=w519, y="Resize") -> (x != y?=w517:bool)
            n151 = call <vilib>:"Adjust Cursor Y Position to Maintain Label Placement.vi"("Refnums for Resizing and Alignment"=w520, "Display State In"=w524) -> ("Display State Out"=w526:T2)  [unwired: 9 in]
            n152 = call <vilib>:"Set Colors.vi"("Refnums"=w520, "Display State In"=w526) -> ("Display State Out"=w521:T2)  [unwired: 9 in]
          }
        }
        n153 = case shown="False" w490 {
          selector: w490 -> [_ w507]
          tunnel: [w503 w512] -> w502
          tunnel: w501 -> [w505 w511]
          tunnel: [w505 w510] -> w500
          tunnel: w494 -> [w503 w509]
          tunnel: w492 -> [_ w508]
          tunnel: [w504 w506] -> w489
          tunnel: w488 -> [w504 w506]
          frame False {
          }
          frame True {
            n154 = Bundle By Name(cluster=w509, "Action Name"=w508, "Data Changed?"=w507) -> (w512:T1)
            n155 = Generate User Event(user event=w511, event data cluster=w507) -> (user event out=w510:refnum<user-event>)  [unwired: 2 in, 1 out]
          }
        }
        n156 = call <vilib>:"Generate Matching User Event.vi"("event"=w492, "Display State in"=w496) -> ("Display State out"=w497:T2)  [unwired: 8 in, 1 out]
      }
      event Data Change; User Event {
        # "A value was written to the XControl's terminal, local or value property.\nUpdate the appearance in response to data change."
        n157 = event-data() -> ()  [unwired: 1 in, 1 out]
        n158 = flat-sequence {
          tunnel: w535 -> [w548]
          tunnel: w536 -> [w547]
          tunnel: w537 -> [w546]
          tunnel: [w545] -> w534
          tunnel: [w547] -> w533
          tunnel: [w548] -> w532
          tunnel: w528 -> [w543]
          tunnel: [w542] -> w527
          tunnel: w534 -> [w555]
          tunnel: w533 -> [w552]
          tunnel: w532 -> [w554]
          tunnel: [w549] -> w538
          tunnel: [w553] -> w531
          tunnel: [w551] -> w530
          tunnel: w527 -> [w550]
          frame #0 {
            # "write data to graph"
            n159 = To Single Precision Float(number=w548) -> (single precision float=→"Waveform Graph":waveform(sgl)[])
            n160 = Unbundle By Name(w543) -> ("Action Name"=w542:string)
            n161 = call <vilib>:"Generate Matching User Event.vi"("event"=T8 "Data Change", "Display State in"=w546) -> ("Display State out"=w545:T2)  [unwired: 8 in, 1 out]
          }
          frame #1 {
            # "cursors"
            n162 = case shown="Default" w550 {
              tunnel: w555 -> [w558 w564]
              tunnel: w554 -> [w556 w561]
              tunnel: [w558 w563] -> w553
              tunnel: w552 -> [w559 w562]
              tunnel: [w559 w562] -> w551
              tunnel: [w556 w560] -> w549
              frame "APP_SC_CLEAR_GRAPH" {
                n163 = local write "Cursor Table"(string[][] [[" "]] ("Cursor Table")) -> ()
              }
              frame Default {
                n164 = call <vilib>:"Get Cursor Values from Data.vi"("waveforms"=w561, "Refnums for FP Objects"=w562, "Display State In"=w564) -> ("Display State Out"=w563:T2, "waveforms"=w560:T6)  [unwired: 4 in, 3 out]
              }
            }
          }
        }
      }
      event Direction Change {
        # "The direction of the XControl changed from a control to an indicator or vice versa. Update the appearance accordingly."
        n165 = event-data() -> ()  [unwired: 1 in, 4 out]
        n166 = Unbundle By Name(w567) -> ("Splitters.Locked"=w573:refnum<vi>)
        n167 = Unbundle By Name(w576) -> ("Refnum"=w569:refnum<vi>)
        n168 = property class="Splitter"(reference=w573, "Colors"=T9 {"Foreground Color"=16777216, "Background Color"=16777216}) -> ()  [unwired: 1 in, 2 out]
        n169 = property class="Ctl"(reference=w569, "SyncDisp"=TRUE ("Synchronous Display")) -> ()  [unwired: 1 in, 2 out]
      }
      event Exec State Change {
        # "The VI owning the XControl changed from Edit Mode  to Run Mode or vice versa.\nUpdate the appearance accordingly."
        # "Handle Edit Mode & Run Mode case differently"
        n170 = event-data() -> ()  [unwired: 1 in, 4 out]
        n171 = Unbundle By Name(w584) -> ()  [unwired: 1 out]
      }
    }
  }
  "Display State Out" <- w5
  "Data Out" <- w7
  "Action" <- w2
